vi "Set  ActiveCell by Row Or Column.vi"(8 "error in (no error)":errorcluster caption="错误输入（无错误）", 9 "Option":T1(ring), 10 "N":i32, 11 "Table Ref In":refnum<vi>) -> (0 "error out":errorcluster caption="错误输出", 2 "ActiveCell Out":T2, 3 "Table Ref Out":refnum<vi>)   [LabVIEW 2013, in "Table Tool.lvlib"]
uses:
  Table Tool.lvlib
  <vilib>/Utility/miscctls.llb/LVRowAndColumnTypeDef.ctl
  Custum Type/GetOrSet.ctl
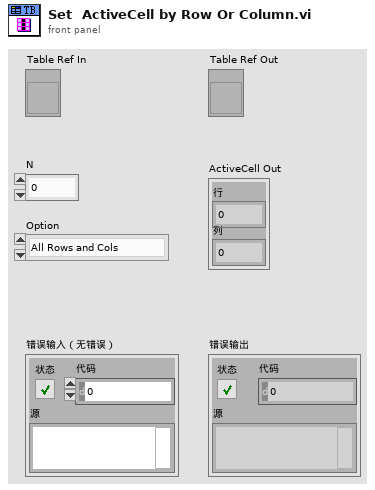
[diagram p1: front panel]
types:
  T1 = enum16{"All Rows and Cols", "Row Head", "Col Head", "N Row", "N Col"}
  T2 = typedef "LVRowAndColumnTypeDef.ctl" = cluster{"Row":i32, "Column":i32}
  T3 = typedef "Table Tool.lvlib/GetOrSet.ctl" = enum16{"Get", "Set"}
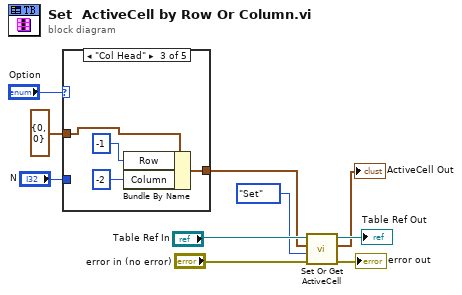
[diagram p0: block diagram]
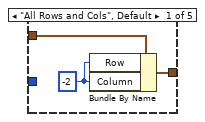
[diagram p2: hidden frame]
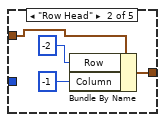
[diagram p3: hidden frame]
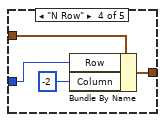
[diagram p4: hidden frame]
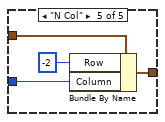
[diagram p5: hidden frame]
diagram:
  n1 = case shown="\"Col Head\"" "Option" {
    tunnel: T2 {"Row"=0, "Column"=0} ("ActiveCell In") -> [w13 w15 w20 w25 w29]
    tunnel: [w11 w14 w21 w22 w26] -> w3
    tunnel: "N" -> [_ _ _ w24 w28]
    frame "All Rows and Cols", Default {
      w12 = -2 ("Row")
      n2 = Bundle By Name(cluster=w13, "Row"=w12, "Column"=w12) -> (w11:T2)
    }
    frame "Row Head" {
      n3 = Bundle By Name(cluster=w15, "Row"=-2, "Column"=-1) -> (w14:T2)
    }
    frame "Col Head" {
      n4 = Bundle By Name(cluster=w20, "Row"=-1, "Column"=-2) -> (w21:T2)
    }
    frame "N Row" {
      n5 = Bundle By Name(cluster=w25, "Row"=w24, "Column"=-2) -> (w22:T2)
    }
    frame "N Col" {
      n6 = Bundle By Name(cluster=w29, "Row"=-2, "Column"=w28) -> (w26:T2)
    }
  }
  n7 = call "Set Or Get ActiveCell.vi"("error in (no error)"="error in (no error)", "Mode"=GetOrSet."Set", "ActiveCell In"=w3, "Table Ref In"="Table Ref In") -> ("error out"=→"error out":errorcluster, "ActiveCell Out"=→"ActiveCell Out":T2, "Table Ref Out"=→"Table Ref Out":refnum<vi>)  [unwired: 5 in]
